vi "Generate Differential Drive Trajectory from Control Vectors.vi"(8 "error in (no error)":errorcluster, 9 "Constraints":T5={"maxVoltage"=10.0, "maxVelocity"=5.0, "maxAccel"=10.0}, 10 "Constants":T6={"ks"=0.2, "kv"=0.18, "ka"=0.1, "trackwidth"=1.0}, 11 "Control Vectors":T4(array[cluster])) -> (0 "error out":errorcluster, 2 "Total Time Seconds":dbl, 3 "states":T7[](array[typedef]))   [LabVIEW 2019]
uses:
  Typedef/Trajectory State.ctl
  Geometry/Typedef/Pose2d.ctl
  Geometry/Typedef/Translation2d.ctl
  Geometry/Typedef/Rotation2d.ctl
  Typedef/Differential Drive Constants.ctl
  Typedef/Differential Drive Constraints.ctl
  <vilib>/Analysis/coordinate.llb/2D Cartesian Coordinate Rotation (Scalar).vi
  <vilib>/Analysis/NI_AALPro.lvlib
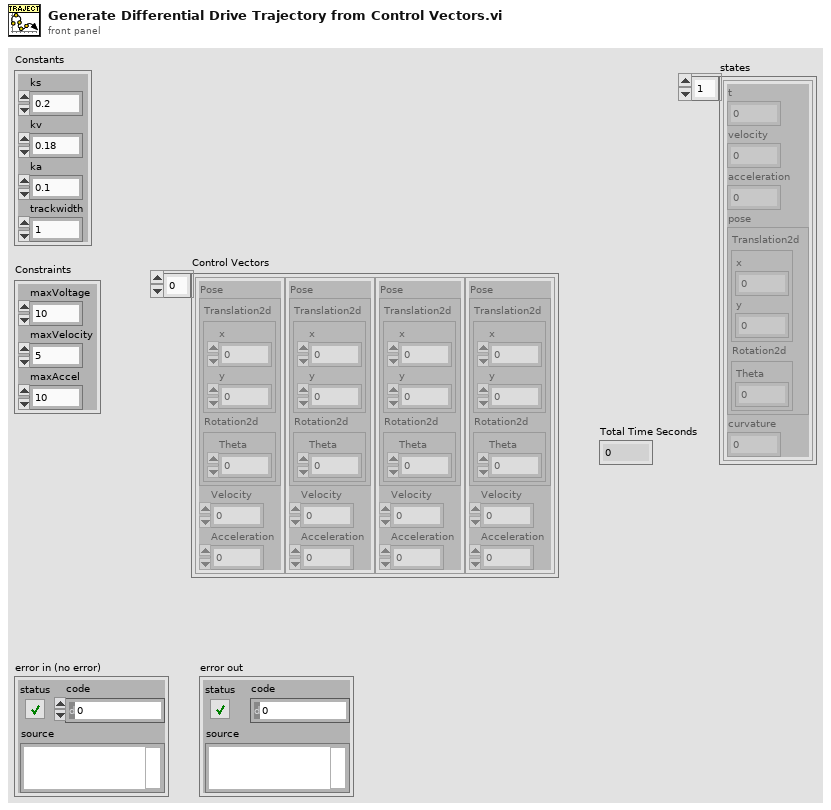
[diagram p1: front panel]
types:
  T1 = typedef "Pose2d.ctl" = cluster{"Translation2d":T2, "Rotation2d":T3}
  T2 = typedef "Translation2d.ctl" = cluster{"x":dbl, "y":dbl}
  T3 = typedef "Rotation2d.ctl" = cluster{"Theta":dbl}
  T4 = cluster{"Pose":T1, "Velocity":dbl, "Acceleration":dbl}[]
  T5 = typedef "Differential Drive Constraints.ctl" = cluster{"maxVoltage":dbl, "maxVelocity":dbl, "maxAccel":dbl}
  T6 = typedef "Differential Drive Constants.ctl" = cluster{"ks":dbl, "kv":dbl, "ka":dbl, "trackwidth":dbl}
  T7 = typedef "Trajectory State.ctl" = cluster{"t":dbl, "velocity":dbl, "acceleration":dbl, "pose":T1, "curvature":dbl}
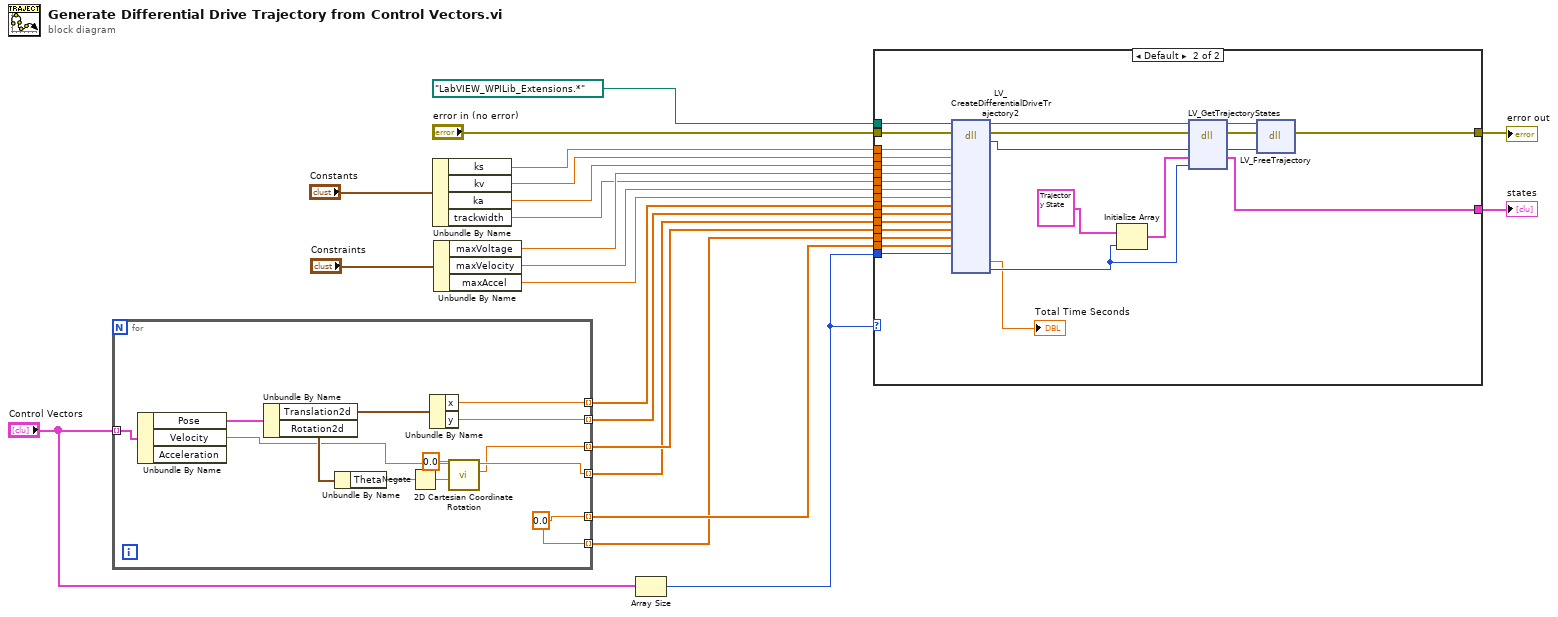
[diagram p0: block diagram]
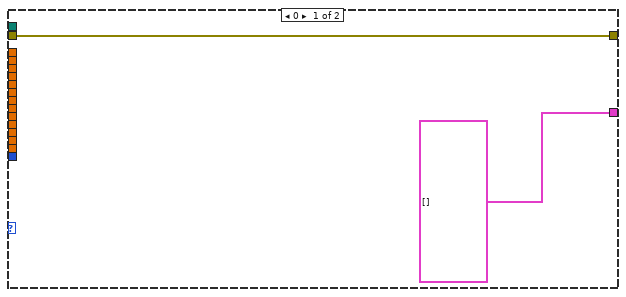
[diagram p2: hidden frame]
diagram:
  n1 = for {
    tunnel: "Control Vectors" -> [w34] mode=indexing
    tunnel: [w31] -> w9 mode=indexing
    tunnel: [w30] -> w8 mode=indexing
    tunnel: [w23] -> w7 mode=indexing
    tunnel: [w24] -> w6 mode=indexing
    tunnel: [w22] -> w5 mode=indexing
    tunnel: [w22] -> w4 mode=indexing
    w22 = 0.0 ("y")
    n2 = Unbundle By Name(w34) -> ("Pose"=w33:T1, "Velocity"=w26:dbl)  [unwired: 1 out]
    n3 = Unbundle By Name(w33) -> ("Translation2d"=w32:T2, "Rotation2d"=w29:T3)
    n4 = Unbundle By Name(w29) -> ("Theta"=w28:dbl)
    n5 = Negate(x=w28) -> (-x=w27:dbl)
    n6 = Unbundle By Name(w32) -> ("x"=w31:dbl, "y"=w30:dbl)
    n7 = call-poly <vilib>:"2D Cartesian Coordinate Rotation.vi"("theta"=w27, "y"=0.0, "x"=w26) -> ("y out"=w23:dbl, "x out"=w24:dbl)  [unwired: 6 in, 1 out]
  }
  n8 = Unbundle By Name("Constants") -> ("ks"=w13:dbl, "kv"=w14:dbl, "ka"=w15:dbl, "trackwidth"=w16:dbl)
  n9 = Unbundle By Name("Constraints") -> ("maxVoltage"=w18:dbl, "maxVelocity"=w19:dbl, "maxAccel"=w20:dbl)
  n10 = Array Size(array="Control Vectors") -> (size(s)=w1:i32)
  n11 = case shown="Default" w1 {
    tunnel: path "LabVIEW_WPILib_Extensions.*" ("path in") -> [_ w60]
    tunnel: w20 -> [_ w59]
    tunnel: w19 -> [_ w58]
    tunnel: w18 -> [_ w57]
    tunnel: w16 -> [_ w56]
    tunnel: w15 -> [_ w55]
    tunnel: w14 -> [_ w54]
    tunnel: w13 -> [_ w53]
    tunnel: w1 -> [_ w52]
    tunnel: "error in (no error)" -> [w35 w45]
    tunnel: w9 -> [_ w44]
    tunnel: w8 -> [_ w43]
    tunnel: w7 -> [_ w42]
    tunnel: w6 -> [_ w41]
    tunnel: w5 -> [_ w40]
    tunnel: w4 -> [_ w39]
    tunnel: [T7[] [] ("states") w38] -> w3
    tunnel: [w35 w37] -> w2
    frame 0 {
    }
    frame Default {
      n12 = dll-call lib="?" fn="LV_CreateDifferentialDriveTrajectory2"(path in=w60, error in=w45, "ks"=w53, "kv"=w54, "ka"=w55, "maxVoltage"=w57, "trackwidth"=w56, "maxVelocity"=w58, "maxAccel"=w59, "position_vector_x"=w44, "position_vector_y"=w43, "velocity_vector_x"=w41, "velocity_vector_y"=w42, "acceleration_vector_x"=w39, "acceleration_vector_y"=w40, "numPoints"=w52) -> (path out=w61:path, error out=w63:errorcluster, "return type"=w47:u64, "totalTimeSeconds"=→"Total Time Seconds":dbl, "trajectorySize"=w49:u32)  [unwired: 17 in]
      n13 = Initialize Array(T7 {"t"=0.0, "velocity"=0.0, "acceleration"=0.0, "pose"={"Translation2d"={"x"=0.0, "y"=0.0}, "Rotation2d"={"Theta"=0.0}}, "curvature"=0.0}, w49) -> (w48:T7[])
      n14 = dll-call lib="?" fn="LV_GetTrajectoryStates"(path in=w61, error in=w63, "handle"=w47, "states"=w48, "bufsize"=w49) -> (path out=w62:path, error out=w64:errorcluster, "handle"=w51:u64, "states"=w38:T7[])  [unwired: 3 in]
      n15 = dll-call lib="?" fn="LV_FreeTrajectory"(path in=w62, error in=w64, "handle"=w51) -> (error out=w37:errorcluster)  [unwired: 3 in, 1 out]
    }
  }
  "states" <- w3
  "error out" <- w2
